vi "Supports Folder.vi"(8 "error in (no error)":errorcluster, 10 "Path":path, 11 "GitPackage in":refnum<class "GitPackage.lvclass">) -> (0 "error out":errorcluster, 1 "Root Folder":path, 2 "Supported":bool, 3 "GitPackage out":refnum<class "GitPackage.lvclass">)   [LabVIEW 2020, in "GPack.lvlib" / "GitPackage.lvclass"]
uses:
  GitPackage.lvclass
  <vilib>/Hampel Software Engineering/Git API/Git API/GIT-api.lvclass
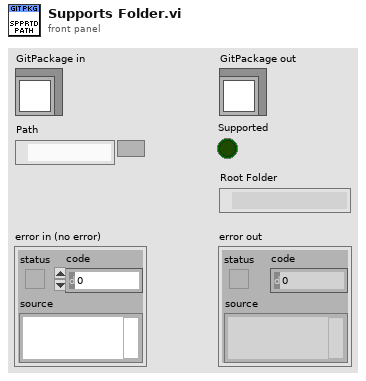
[diagram p1: front panel]
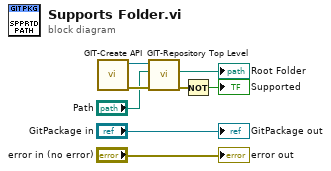
[diagram p0: block diagram]
diagram:
  n1 = call <vilib>:"GIT-Create API.vi"() -> ("error out"=w8:errorcluster, "git-api out"=w4:refnum<class "GIT-api.lvclass">)  [unwired: 10 in]
  n2 = call <vilib>:"GIT-Repository Top Level.vi"("error in"=w8, "Current Path"="Path", "git-api in"=w4) -> ("error out"=w2:errorcluster, "Repo Top Level Path"=→"Root Folder":path)  [unwired: 6 in, 1 out]
  n3 = Not(x=w2) -> (.not. x?=→"Supported":bool)
  "error out" <- "error in (no error)"
  "GitPackage out" <- "GitPackage in"
